vi "Set Session.vi"(8 "error in (no error)":errorcluster, 10 "Session":refnum<k21>, 11 "XNET Base CFG in":refnum<class "XNET Base CFG.lvclass">) -> (0 "error out":errorcluster, 3 "XNET Base CFG out":refnum<class "XNET Base CFG.lvclass">)   [LabVIEW 2023, in "XNET Base CFG.lvclass"]
uses:
  XNET Base CFG.lvclass
  XNET Base CFG.lvclass/XNET Base CFG.ctl
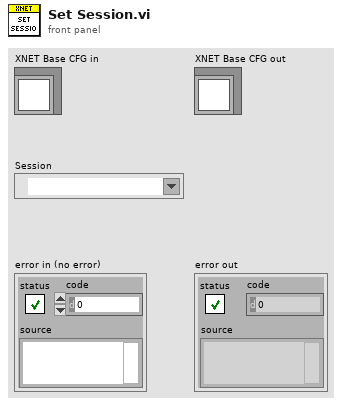
[diagram p1: front panel]
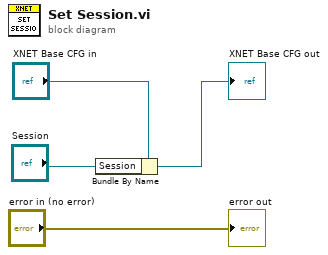
[diagram p0: block diagram]
diagram:
  n1 = Bundle By Name(cluster="XNET Base CFG in", "Session"="Session") -> (→"XNET Base CFG out":refnum<class "XNET Base CFG.lvclass">)
  "error out" <- "error in (no error)"
